vi "_Add Cell.vi"(8 "error in":errorcluster, 10 "Cell Address":string, 11 "Row in":refnum<k24>) -> (0 "error out":errorcluster, 2 "Cell":refnum<k24>, 3 "Row out":refnum<k24>)   [LabVIEW 2021, in "Open Xml.lvlib"]
uses:
  Open Xml.lvlib
  D:/git/Open-Xml-LabVIEW/dll/DocumentFormat.OpenXml.dll
  dll/DocumentFormat.OpenXml.dll
  D:/git/Open-Xml-LabVIEW/dll/DocumentFormat.OpenXml.Framework.dll
  dll/DocumentFormat.OpenXml.Framework.dll
  D:/git/Open-Xml-LabVIEW/dll/OpenXmlGenericsWrapper.dll
  dll/OpenXmlGenericsWrapper.dll
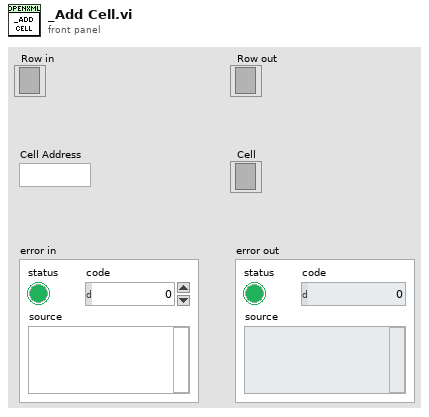
[diagram p1: front panel]
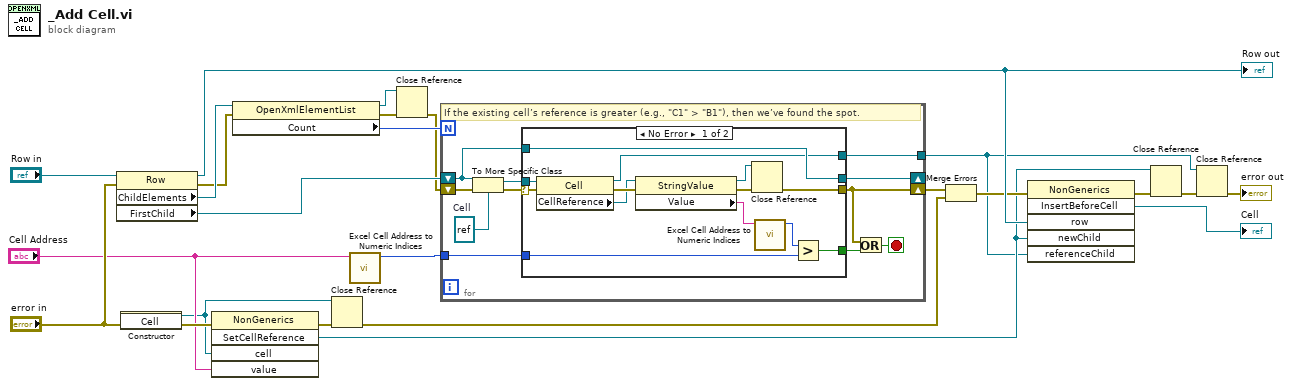
[diagram p0: block diagram]
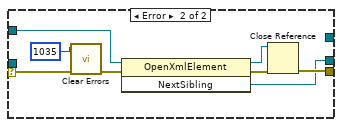
[diagram p2: hidden frame]
diagram:
  n1 = property class="Row"(reference="Row in", error in="error in") -> (reference out=w9:refnum<k24>, error out=w19:errorcluster, "ChildElements"=w23:refnum<k24>, "FirstChild"=w21:refnum<k24>)
  "Row out" <- w9
  n2 = constructor class="Cell"(error in="error in") -> (reference out=w3:refnum<k24>, error out=w17:errorcluster)  [unwired: 2 in, 1 out]
  n3 = invoke class="NonGenerics" method="SetCellReference"(error in=w17, "cell"=w3, "value"="Cell Address") -> (error out=w16:errorcluster, "SetCellReference"=w5:refnum<k24>)  [unwired: 2 in, 3 out]
  n4 = property class="OpenXmlElementList"(reference=w23, error in=w19) -> (reference out=w13:refnum<k24>, error out=w20:errorcluster, "Count"=w22:i32)
  n5 = Close Reference(reference=w3, error in (no error)=w16) -> (error out=w4:errorcluster)
  n6 = call "Excel Cell Address to Numeric Indices.vi"("Cell Name"="Cell Address") -> ("Column Number"=w18:i32)  [unwired: 9 in, 1 out]
  n7 = Close Reference(reference=w13, error in (no error)=w20) -> (error out=w14:errorcluster)
  n8 = for {
    N: w22 -> [_]
    tunnel: w18 -> [w28]
    shift-right: [w26] -> _
    shift-left: w21 -> [w29]
    tunnel: [w25] -> w2
    shift-right: [w32] -> w12
    shift-left: w14 -> [w33]
    stop <- w31 stop-if-true
    w34 = refnum<k24> refnum  # Cell
    # "If the existing cell’s reference is greater (e.g., \"C1\" > \"B1\"), then we’ve found the spot."
    n9 = To More Specific Class(target class=w34, reference=w29, error in=w33) -> (specific class reference=w30:refnum<k24>, error out=w35:errorcluster)
    n10 = case shown="No Error" w35 {
      selector: w35 -> [w48 w56]
      tunnel: [w37 w50] -> w32
      tunnel: w30 -> [w47 _]
      tunnel: w29 -> [w39 w53]
      tunnel: w28 -> [w43 _]
      tunnel: [w40 _] -> w27
      tunnel: [w39 w49] -> w26
      tunnel: [w38 _] -> w25
      frame No Error {
        n11 = property class="Cell"(reference=w47, error in=w48) -> (reference out=w38:refnum<k24>, error out=w46:errorcluster, "CellReference"=w45:refnum<k24>)
        n12 = property class="StringValue"(reference=w45, error in=w46) -> (reference out=w36:refnum<k24>, error out=w42:errorcluster, "Value"=w44:string)
        n13 = Close Reference(reference=w36, error in (no error)=w42) -> (error out=w37:errorcluster)
        n14 = call "Excel Cell Address to Numeric Indices.vi"("Cell Name"=w44) -> ("Column Number"=w41:i32)  [unwired: 9 in, 1 out]
        n15 = Greater?(x=w41, y=w43) -> (0:w40:bool)
      }
      frame Error {
        n16 = call <vilib>:"Clear Errors.vi"("error in (no error)"=w56, "specific error code to clear (0: all)"=1035) -> ("error out"=w54:errorcluster)  [unwired: 4 in, 1 out]
        n17 = invoke class="OpenXmlElement" method="NextSibling"(reference=w53, error in=w54) -> (reference out=w52:refnum<k24>, error out=w51:errorcluster, "NextSibling"=w49:refnum<k24>)  [unwired: 1 in]
        n18 = Close Reference(reference=w52, error in (no error)=w51) -> (error out=w50:errorcluster)
      }
    }
    n19 = Or(x=w32, y=w27) -> (x .or. y?=w31:bool)
  }
  n20 = Merge Errors(w12, w4) -> (w8:errorcluster)
  n21 = invoke class="NonGenerics" method="InsertBeforeCell"(error in=w8, "row"=w9, "newChild"=w5, "referenceChild"=w2) -> (error out=w11:errorcluster, "InsertBeforeCell"=→"Cell":refnum<k24>)  [unwired: 2 in, 4 out]
  n22 = Close Reference(reference=w5, error in (no error)=w11) -> (error out=w6:errorcluster)
  n23 = Close Reference(reference=w2, error in (no error)=w6) -> (error out=→"error out":errorcluster)
